vi "Empty Directory.vi"(7 "Delete Files Without Prompt? (F)":bool, 8 "Error In":errorcluster, 11 "Directory":path=path "D:/workspace/revert/working directory") -> (0 "Error Out":errorcluster, 2 "Aborted?":bool, 3 "Duplicate Path":path)   [LabVIEW 2020, in "LMH-Toolbox.lvlib"]
doc: "Delete all files within a directory (but leave the empty diretory). The user will be prompted if files are in use and cannot be deleted."
uses:
  LMH-Toolbox.lvlib
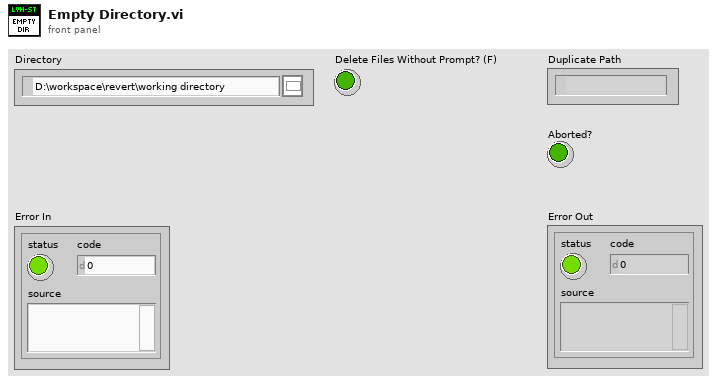
[diagram p1: front panel]
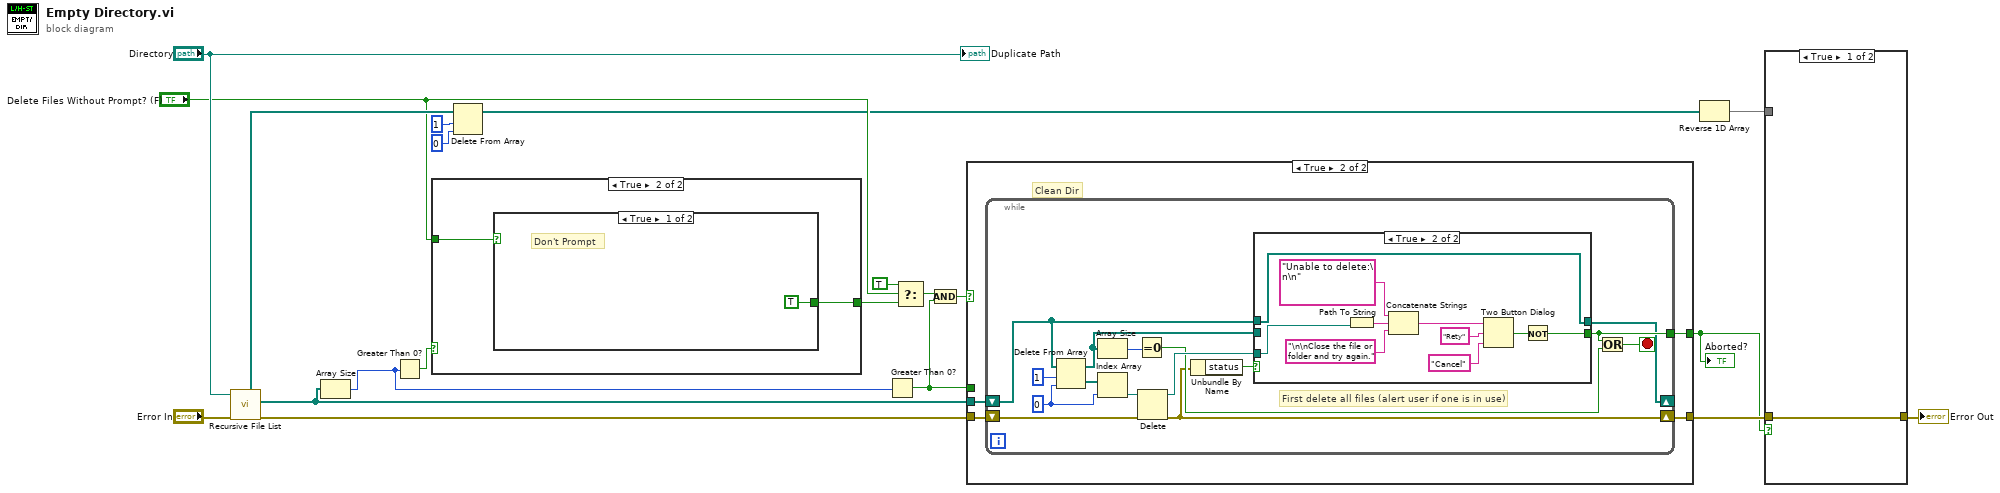
[diagram p0: block diagram]
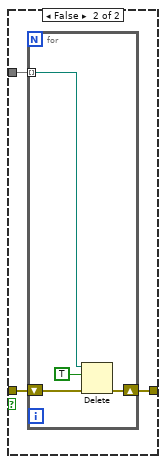
[diagram p2: hidden frame]
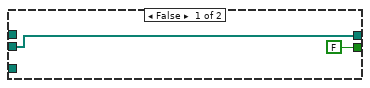
[diagram p4: hidden frame]
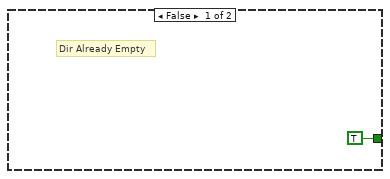
[diagram p5: hidden frame]
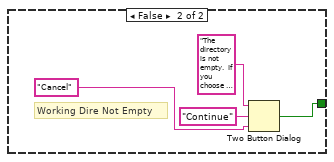
[diagram p6: hidden frame]
diagram:
  n1 = call <vilib>:"Recursive File List.vi"("error in (no error)"="Error In", "Folder Path"="Directory") -> ("error out"=w17:errorcluster, "All Files in Dir"=w15:path[], "All Folders"=w10:path[])  [unwired: 5 in, 2 out]
  n2 = Array Size(array=w15) -> (size(s)=w1:i32)
  n3 = Greater Than 0?(x=w1) -> (x > 0?=w20:bool)
  n4 = case shown="True" w20 {
    tunnel: [TRUE ("T button?") w23] -> w19
    tunnel: "Delete Files Without Prompt? (F)" -> [_ w22]
    frame False {
      # "Dir Already Empty"
    }
    frame True {
      n5 = case shown="True" w22 {
        tunnel: [TRUE ("T button?") w25] -> w23
        frame True {
          # "Don't Prompt"
        }
        frame False {
          # "Working Dire Not Empty"
          n6 = Two Button Dialog(message="The directory is not empty.  If you choose to continue all files and folders in the directory will be lost.", 1:"Cancel" ("T button name (\"OK\")"), 2:"Continue" ("T button name (\"OK\")")) -> (T button?=w25:bool)
        }
      }
    }
  }
  n7 = Delete From Array(array=w10, length=1, index=0) -> (array with subset deleted=w3:path[])  [unwired: 1 out]
  n8 = Greater Than 0?(x=w1) -> (x > 0?=w5:bool)
  n9 = Select(t=TRUE, s="Delete Files Without Prompt? (F)", f=w19) -> (s? t:f=w7:bool)
  n10 = And(x=w7, y=w5) -> (x .and. y?=w6:bool)
  n11 = case shown="True" w6 {
    tunnel: w17 -> [w30 w33]
    tunnel: [w30 w31] -> w13
    tunnel: [w29 w32] -> w11
    tunnel: w15 -> [_ w34]
    tunnel: w5 -> [w29 _]
    frame False {
    }
    frame True {
      # "Clean Dir"
      n12 = while {
        shift-right: [w38] -> w31
        shift-left: w33 -> [w49]
        shift-right: [w36] -> _
        shift-left: w34 -> [w35]
        tunnel: [w39] -> w32
        stop <- w41 stop-if-true
        w44 = 0 ("index")
        # "First delete all files (alert user if one is in use)"
        n13 = Delete From Array(array=w35, length=1, index=w44) -> (deleted portion=w45:path[], array with subset deleted=w37:path[])
        n14 = Array Size(array=w37) -> (size(s)=w47:i32)
        n15 = Index Array(array=w45, index=w44) -> (element=w43:path)
        n16 = Equal To 0?(x=w47) -> (x = 0?=w40:bool)
        n17 = Delete(path (use dialog)=w43, error in=w49) -> (deleted path=w42:path, error out=w38:errorcluster)  [unwired: 3 in, 1 out]
        n18 = Unbundle By Name(w38) -> ("status"=w48:bool)
        n19 = case shown="True" w48 {
          tunnel: w42 -> [_ w55]
          tunnel: [FALSE w53] -> w39
          tunnel: w37 -> [w50 _]
          tunnel: [w50 w52] -> w36
          tunnel: w35 -> [_ w52]
          frame False {
          }
          frame True {
            n20 = Path To String(path=w55) -> (string=w57:string)
            n21 = Concatenate Strings("Unable to delete:\n\n" ("message"), w57, "\n\nClose the file or folder and try again." ("message")) -> (w56:string)
            n22 = Two Button Dialog(message=w56, 1:"Cancel" ("T button name (\"OK\")"), 2:"Rety" ("T button name (\"OK\")")) -> (T button?=w54:bool)
            n23 = Not(x=w54) -> (.not. x?=w53:bool)
          }
        }
        n24 = Or(x=w39, y=w40) -> (x .or. y?=w41:bool)
      }
    }
  }
  "Aborted?" <- w11
  n25 = Reverse 1D Array(array=w3) -> (reversed array=w2:path[])
  n26 = case shown="True" w11 {
    tunnel: w13 -> [w62 w64]
    tunnel: [w62 w65] -> w12
    tunnel: w2 -> [_ w63]
    frame True {
    }
    frame False {
      n27 = for {
        tunnel: w63 -> [w67] mode=indexing
        shift-right: [w69] -> w65
        shift-left: w64 -> [w66]
        n28 = Delete(path (use dialog)=w67, entire hierarchy (F)=TRUE, error in=w66) -> (error out=w69:errorcluster)  [unwired: 2 in, 2 out]
      }
    }
  }
  "Error Out" <- w12
  "Duplicate Path" <- "Directory"
